vi "assets.create.vi"(8 "error in":errorcluster, 9 "nominalDataSourceRid":string, 10 "name":string, 11 "Nominal Client in":refnum<class "Nominal Client.lvclass">) -> (0 "error out":errorcluster, 1 "Response":string, 2 "response":T1, 3 "Nominal Client out":refnum<class "Nominal Client.lvclass">)   [LabVIEW 2020, in "Nominal Client.lvclass"]
doc: "Creates a new asset."
uses:
  Nominal Client.lvclass
  Nominal Client.lvclass/Nominal Client.ctl
  301638a4-f299-4835-8683-15cfc56d6fd6.vi
  28804fc9-aee6-4b6e-ba11-1ba961eefadd.vi
  <vilib>/JDP Science/JSONtext/JSONtext.lvlib
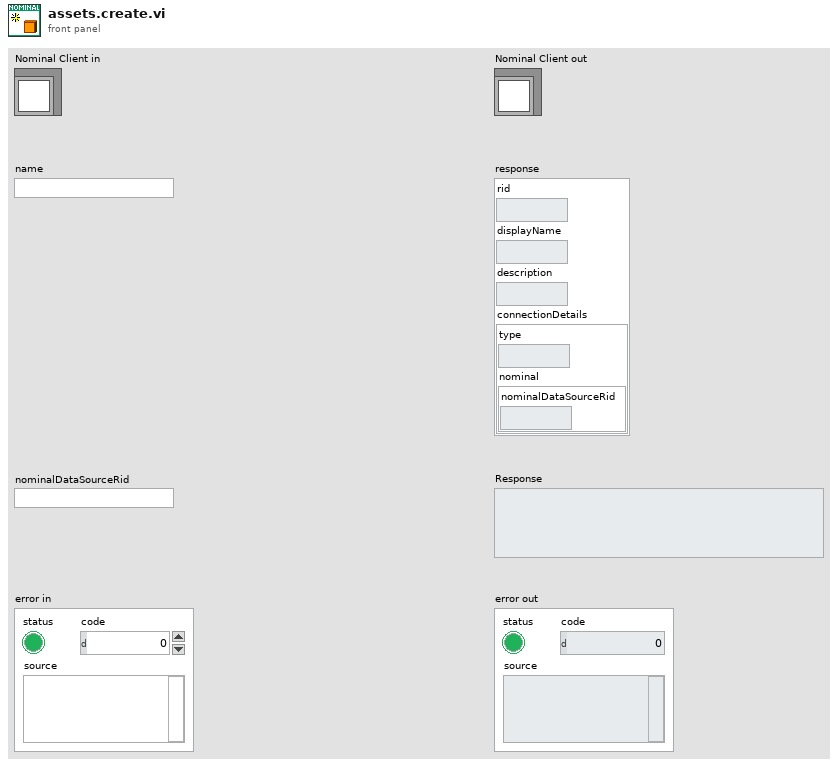
[diagram p1: front panel]
types:
  T1 = cluster{"rid":string, "displayName":string, "description":string, "connectionDetails":cluster{"type":string, "nominal":cluster{"nominalDataSourceRid":string}}}
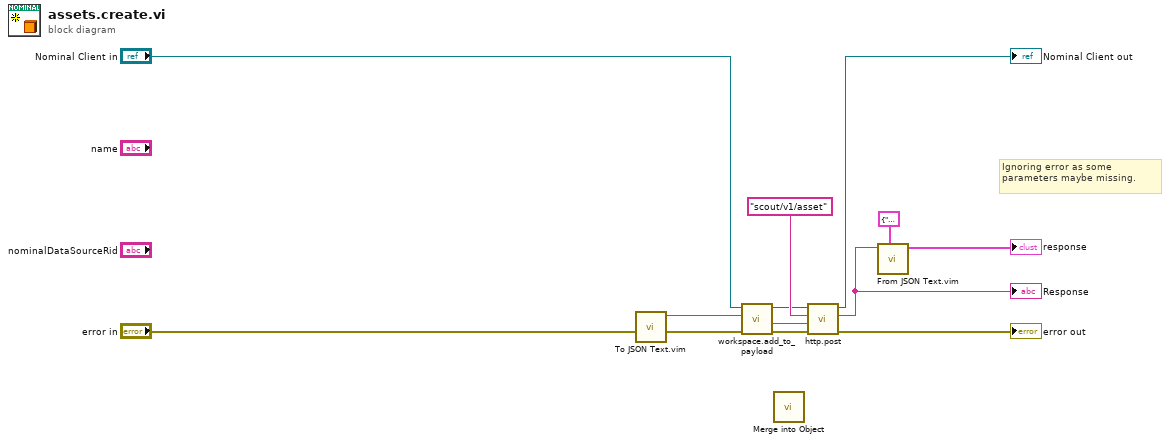
[diagram p0: block diagram]
diagram:
  # "Ignoring error as some parameters maybe missing."
  n1 = call "To JSON Text.vim"("error in (no error)"="error in") -> ("error out"=w1:errorcluster, "<JSON>"=w2:string)  [unwired: 9 in]
  n2 = call "workspace.add_to_payload.vi"("error in"=w1, "JSON payload in"=w2, "Nominal Client in"="Nominal Client in") -> ("error out"=w6:errorcluster, "JSON payload out"=w4:string, "Nominal Client out"=w5:refnum<class "Nominal Client.lvclass">)  [unwired: 6 in]
  n3 = call <vilib>:"Merge into Object.vi"() -> ()  [unwired: 9 in, 2 out]
  n4 = call "http.post.vi"("error in"=w6, "Request body"=w4, "Path"="scout/v1/asset", "Nominal Client in"=w5) -> ("error out"=→"error out":errorcluster, "Response"=w10:string, "Nominal Client out"=→"Nominal Client out":refnum<class "Nominal Client.lvclass">)  [unwired: 4 in, 1 out]
  "Response" <- w10
  n5 = call "From JSON Text.vim"("Data Type and Default Value"=T1 {"rid"="", "displayName"="", "description"="", "connectionDetails"={"type"="", "nominal"={"nominalDataSourceRid"=""}}} ("response"), "JSON"=w10) -> ("Data out"=→"response":T1)  [unwired: 8 in, 1 out]
